vi "Size Mismatch.vi"(7 "error source vi name":string, 8 "error in (no error)":errorcluster, 10 "Pointer b in":refnum<class "Pointer.lvclass">, 11 "Pointer a in":refnum<class "Pointer.lvclass">) -> (0 "error out":errorcluster, 2 "Pointer b out":refnum<class "Pointer.lvclass">, 3 "Pointer a out":refnum<class "Pointer.lvclass">)   [LabVIEW 2016, in "Memory Manager.lvlib" / "Pointer.lvclass"]
uses:
  Pointer.lvclass
  Errors.ctl
  VIs/Source.Write.Scalar.Base10 (U64).vi
  Static Error Handling.lvlib
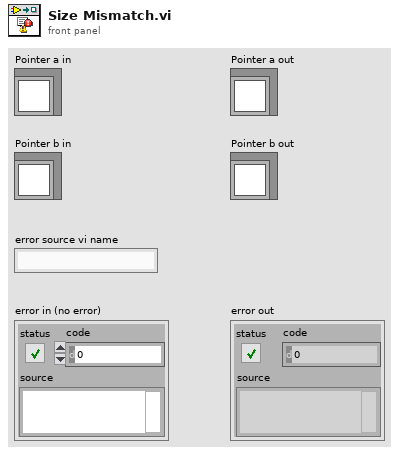
[diagram p1: front panel]
types:
  T1 = typedef "Memory Manager.lvlib/Pointer.lvclass/Errors.ctl" = enum16{"No Error", "Null Pointer", "Out of Bounds", "Buffer Underflow", "Size Mismatch", "Zone"}
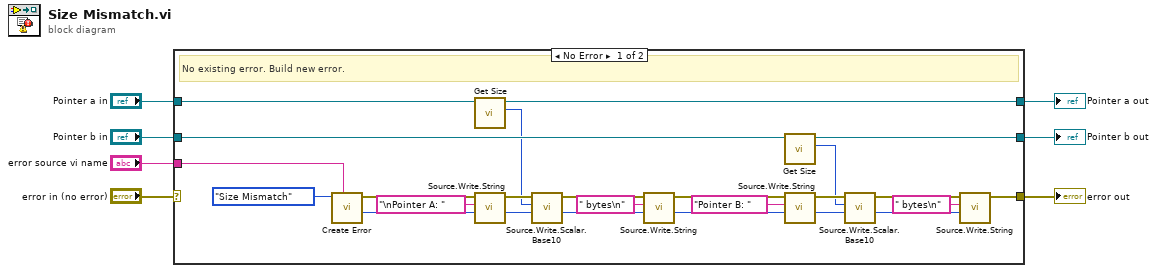
[diagram p0: block diagram]
diagram:
  n1 = case shown="No Error" "error in (no error)" {
    selector: "error in (no error)" -> [_ w35]
    tunnel: [w19 w35] -> w5
    tunnel: "error source vi name" -> [w31 _]
    tunnel: "Pointer b in" -> [w11 w34]
    tunnel: [w10 w34] -> w1
    tunnel: "Pointer a in" -> [w13 w33]
    tunnel: [w12 w33] -> w2
    frame No Error {
      # "No existing error. Build new error."
      n2 = call "Create Error.vi"("source vi name"=w31, "error"=Errors."Size Mismatch") -> ("new offset"=w16:i32, "error out"=w17:errorcluster)  [unwired: 8 in]
      n3 = call "Get Size.vi"("Pointer in"=w13) -> ("size"=w9:u64, "Pointer out"=w12:refnum<class "Pointer.lvclass">)  [unwired: 9 in]
      n4 = call "Source.Write.String.vi"("offset"=w16, "string"="\nPointer A: ", "error in"=w17) -> ("new offset"=w14:i32, "error out"=w15:errorcluster)  [unwired: 7 in]
      n5 = call-poly "Source.Write.Scalar.Base10.vi"("offset"=w14, "value"=w9, "error in"=w15) -> ("new offset"=w28:i32, "error out"=w29:errorcluster)  [unwired: 7 in]
      n6 = call "Source.Write.String.vi"("offset"=w28, "string"=" bytes\n", "error in"=w29) -> ("new offset"=w20:i32, "error out"=w21:errorcluster)  [unwired: 7 in]
      n7 = call "Get Size.vi"("Pointer in"=w11) -> ("size"=w8:u64, "Pointer out"=w10:refnum<class "Pointer.lvclass">)  [unwired: 9 in]
      n8 = call "Source.Write.String.vi"("offset"=w20, "string"="Pointer B: ", "error in"=w21) -> ("new offset"=w25:i32, "error out"=w26:errorcluster)  [unwired: 7 in]
      n9 = call-poly "Source.Write.Scalar.Base10.vi"("offset"=w25, "value"=w8, "error in"=w26) -> ("new offset"=w22:i32, "error out"=w23:errorcluster)  [unwired: 7 in]
      n10 = call "Source.Write.String.vi"("offset"=w22, "string"=" bytes\n", "error in"=w23) -> ("error out"=w19:errorcluster)  [unwired: 7 in, 1 out]
    }
    frame Error {
      # "Incoming error. Pass through."
    }
  }
  "error out" <- w5
  "Pointer a out" <- w2
  "Pointer b out" <- w1
